vi "ChangeInheritanceDialog.vi"(0 "ClassWriter in":refnum<class "ClassWriter.lvclass">, 1 "LvClass":refnum<vi>, 5 "error in (no error)":errorcluster) -> (14 "ClassWriter out":refnum<class "ClassWriter.lvclass">, 15 "BaseClassPath":path, 16 "Cancelled":bool, 19 "error out":errorcluster)   [LabVIEW 2016, in "ClassWriter.lvclass"]
uses:
  <resource>/Framework/Providers/Open_GDS/ClassProviders/Provider_BaseClassInterface/ClassWriter_class/ClassWriter.lvclass
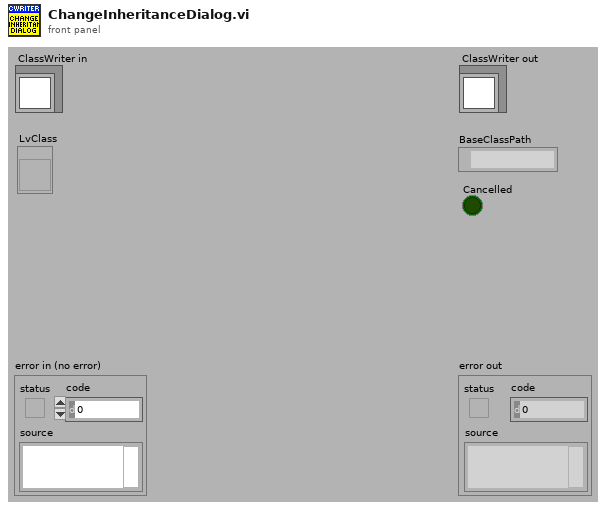
[diagram p1: front panel]
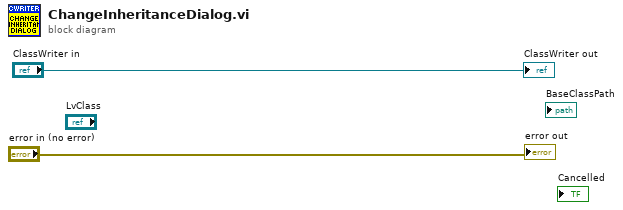
[diagram p0: block diagram]
diagram:
  "error out" <- "error in (no error)"
  "ClassWriter out" <- "ClassWriter in"
